vi "lab2-7-2.vi"() -> ()   [LabVIEW 2020]
panel:
  out "Waveform Graph":waveform(dbl)(graph)
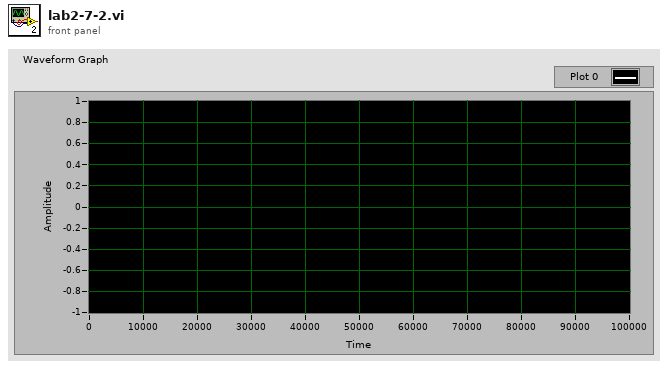
[diagram p1: front panel]
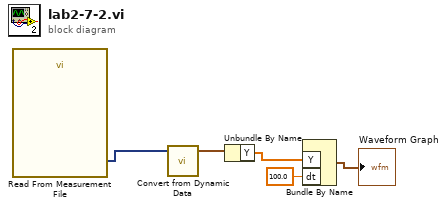
[diagram p0: block diagram]
diagram:
  n1 = call "Read From Measurement File"() -> ("Signals"=w5:dynamicdata)  [unwired: 6 in, 5 out]
  n2 = call "Convert from Dynamic Data"("Dynamic Data Type"=w5) -> ("Waveform"=w4:waveform(dbl))  [unwired: 3 in]
  n3 = Unbundle By Name(w4) -> ("Y"=w3:dbl[])
  n4 = Bundle By Name("Y"=w3, "dt"=100.0) -> (→"Waveform Graph":waveform(dbl))  [unwired: 1 in]
